vi "array2json.vi"(8 "error in (no error)":errorcluster, 11 "Array Refnum in":refnum<vi>) -> (0 "error out":errorcluster, 2 "JSON":string, 3 "Array Refnum out":refnum<vi>)   [LabVIEW 2011, in "JSON.lvlib"]
uses:
  JSON.lvlib
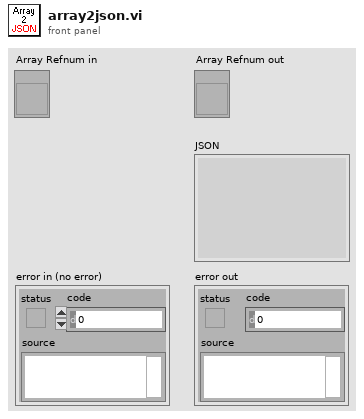
[diagram p1: front panel]
types:
  T1 = typedef "Type Enum.ctl" = enum8{"Void", "I8", "I16", "I32", "I64", "U8", "U16", "U32", "U64", "Single Float", "Double Float", "Extended Float", "Single Complex", "Double Complex", "Extended Complex", "Enum I8 NEVER", "Enum I16 NEVER", "Enum I32 NEVER", "Enum I64 NEVER", "Enum U8", "Enum U16", "Enum U32", "Enum U64", "Single Float With Unit", "Double Float With Unit", "Extended Float With Unit", "Single Complex With Unit", "Double Complex With Unit", "Extended Complex With Unit", "boolU16", "Boolean", "String", "Handle", "Path", "Picture", "C String", "Pascal String", "Tag", "SubString", "Array", "SubArray", "Cluster", "Numeric Cluster", "Variant", "LV Variant", "Measure Data (waveform)", "Refnum", "ExtData", "function", "Typedef", "Poly VI", "bad wire", "LabVIEW Class Instance"}
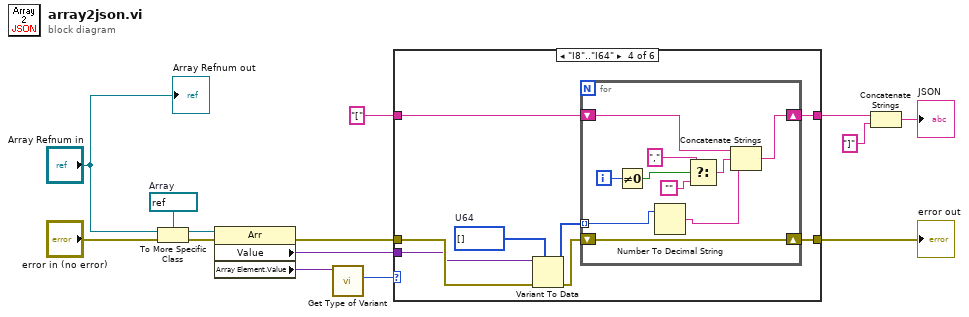
[diagram p0: block diagram]
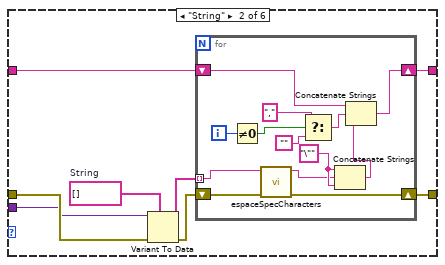
[diagram p3: hidden frame]
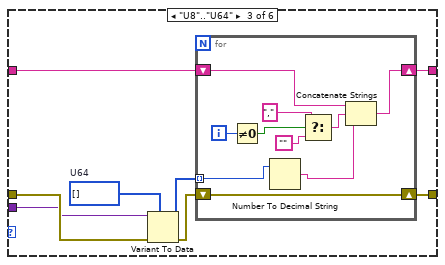
[diagram p4: hidden frame]
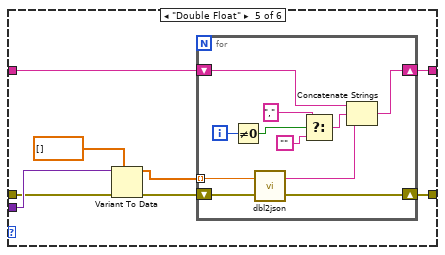
[diagram p5: hidden frame]
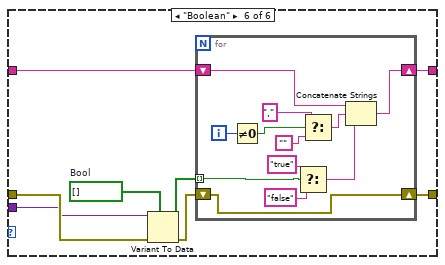
[diagram p6: hidden frame]
diagram:
  w12 = refnum<vi> refnum  # Array
  n1 = To More Specific Class(target class=w12, reference="Array Refnum in", error in="error in (no error)") -> (specific class reference=w11:refnum<vi>, error out=w4:errorcluster)
  n2 = property class="Arr"(reference=w11, error in=w4) -> (error out=w6:errorcluster, "Value"=w7:variant, "Array Element.Value"=w9:variant)  [unwired: 1 out]
  n3 = call <vilib>:"Get Type of Variant.vi"("Data In"=w9) -> ("Type Enum"=w8:T1)  [unwired: 9 in, 1 out]
  n4 = case shown="\"I8\"..\"I64\"" w8 {
    tunnel: w7 -> [_ w22 w43 w61 w81 w98]
    tunnel: w6 -> [w16 w23 w44 w62 w78 w99]
    tunnel: [w16 w21 w42 w60 w76 w97] -> w5
    tunnel: [w15 w20 w41 w59 w75 w96] -> w3
    tunnel: "[" -> [w15 w19 w40 w58 w74 w95]
    frame Default {
    }
    frame "String" {
      w24 = string[] []  # String
      n5 = Variant To Data(error in=w23, type=w24, Variant=w22) -> (data=w17:string[], error out=w18:errorcluster)
      n6 = for {
        shift-right: [w33] -> w20
        shift-left: w19 -> [w32]
        tunnel: w17 -> [w28] mode=indexing
        shift-right: [w29] -> w21
        shift-left: w18 -> [w30]
        i -> [w37]
        w27 = "\"" ("search string")
        n7 = Not Equal To 0?(x=w37) -> (x != 0?=w34:bool)
        n8 = call "espaceSpecCharacters.vi"("error in"=w30, "StringIN"=w28) -> ("error out"=w29:errorcluster, "StringOUT"=w26:string)  [unwired: 8 in]
        n9 = Select(t=",", s=w34, f="") -> (s? t:f=w31:string)
        n10 = Concatenate Strings(w27, w26, w27) -> (w25:string)
        n11 = Concatenate Strings(w32, w31, w25) -> (w33:string)
      }
    }
    frame "U8".."U64" {
      w45 = u64[] []  # U64
      n12 = Variant To Data(error in=w44, type=w45, Variant=w43) -> (data=w38:u64[], error out=w39:errorcluster)
      n13 = for {
        shift-right: [w51] -> w41
        shift-left: w40 -> [w50]
        tunnel: w38 -> [w47] mode=indexing
        shift-right: [w48] -> w42
        shift-left: w39 -> [w48]
        i -> [w55]
        n14 = Not Equal To 0?(x=w55) -> (x != 0?=w52:bool)
        n15 = Number To Decimal String(number=w47) -> (decimal integer string=w46:string)  [unwired: 1 in]
        n16 = Select(t=",", s=w52, f="") -> (s? t:f=w49:string)
        n17 = Concatenate Strings(w50, w49, w46) -> (w51:string)
      }
    }
    frame "I8".."I64" {
      w63 = i64[] []  # U64
      n18 = Variant To Data(error in=w62, type=w63, Variant=w61) -> (data=w56:i64[], error out=w57:errorcluster)
      n19 = for {
        shift-right: [w69] -> w59
        shift-left: w58 -> [w68]
        tunnel: w56 -> [w65] mode=indexing
        shift-right: [w66] -> w60
        shift-left: w57 -> [w66]
        i -> [w73]
        n20 = Not Equal To 0?(x=w73) -> (x != 0?=w70:bool)
        n21 = Number To Decimal String(number=w65) -> (decimal integer string=w64:string)  [unwired: 1 in]
        n22 = Select(t=",", s=w70, f="") -> (s? t:f=w67:string)
        n23 = Concatenate Strings(w68, w67, w64) -> (w69:string)
      }
    }
    frame "Double Float" {
      n24 = Variant To Data(error in=w78, type=dbl[] [], Variant=w81) -> (data=w79:dbl[], error out=w77:errorcluster)
      n25 = for {
        shift-right: [w88] -> w75
        shift-left: w74 -> [w87]
        tunnel: w79 -> [w84] mode=indexing
        shift-right: [w82] -> w76
        shift-left: w77 -> [w83]
        i -> [w92]
        n26 = Not Equal To 0?(x=w92) -> (x != 0?=w89:bool)
        n27 = call "dbl2json.vi"("error in (no error)"=w83, "Numeric"=w84) -> ("error out"=w82:errorcluster, "JSON"=w85:string)
        n28 = Select(t=",", s=w89, f="") -> (s? t:f=w86:string)
        n29 = Concatenate Strings(w87, w86, w85) -> (w88:string)
      }
    }
    frame "Boolean" {
      w100 = bool[] []  # Bool
      n30 = Variant To Data(error in=w99, type=w100, Variant=w98) -> (data=w93:bool[], error out=w94:errorcluster)
      n31 = for {
        shift-right: [w108] -> w96
        shift-left: w95 -> [w107]
        tunnel: w93 -> [w102] mode=indexing
        shift-right: [w105] -> w97
        shift-left: w94 -> [w105]
        i -> [w112]
        n32 = Not Equal To 0?(x=w112) -> (x != 0?=w109:bool)
        n33 = Select(t="true", s=w102, f="false") -> (s? t:f=w101:string)
        n34 = Select(t=",", s=w109, f="") -> (s? t:f=w106:string)
        n35 = Concatenate Strings(w107, w106, w101) -> (w108:string)
      }
    }
  }
  "error out" <- w5
  n36 = Concatenate Strings(w3, "]") -> (→"JSON":string)
  "Array Refnum out" <- "Array Refnum in"
